vi "Remove_Current_Active_Hall_Call.vi"(8 "error in (no error)":errorcluster, 9 "Hall Calls Up/Down in":T1, 10 "Elevator in":T3, 11 "Elevator Fleet in":T10) -> (0 "error out":errorcluster, 1 "Hall Calls Up/Down out":T1, 2 "Elevator out":T3, 3 "Elevator Fleet out":T10)   [LabVIEW 2026]
uses:
  Controls/Elevator_Status.ctl
  Controls/Door_Status_Enum.ctl
  Controls/Occupy_Status.ctl
  Controls/Floor_Status.ctl
  Controls/Motion_Status_Enum.ctl
  Controls/Car_Calls_Status.ctl
  Controls/Hall_Calls_Status.ctl
  Controls/Elevator_Fleet.ctl
  Controls/Hall_Calls.ctl
  Controls/Hall_Floor.ctl
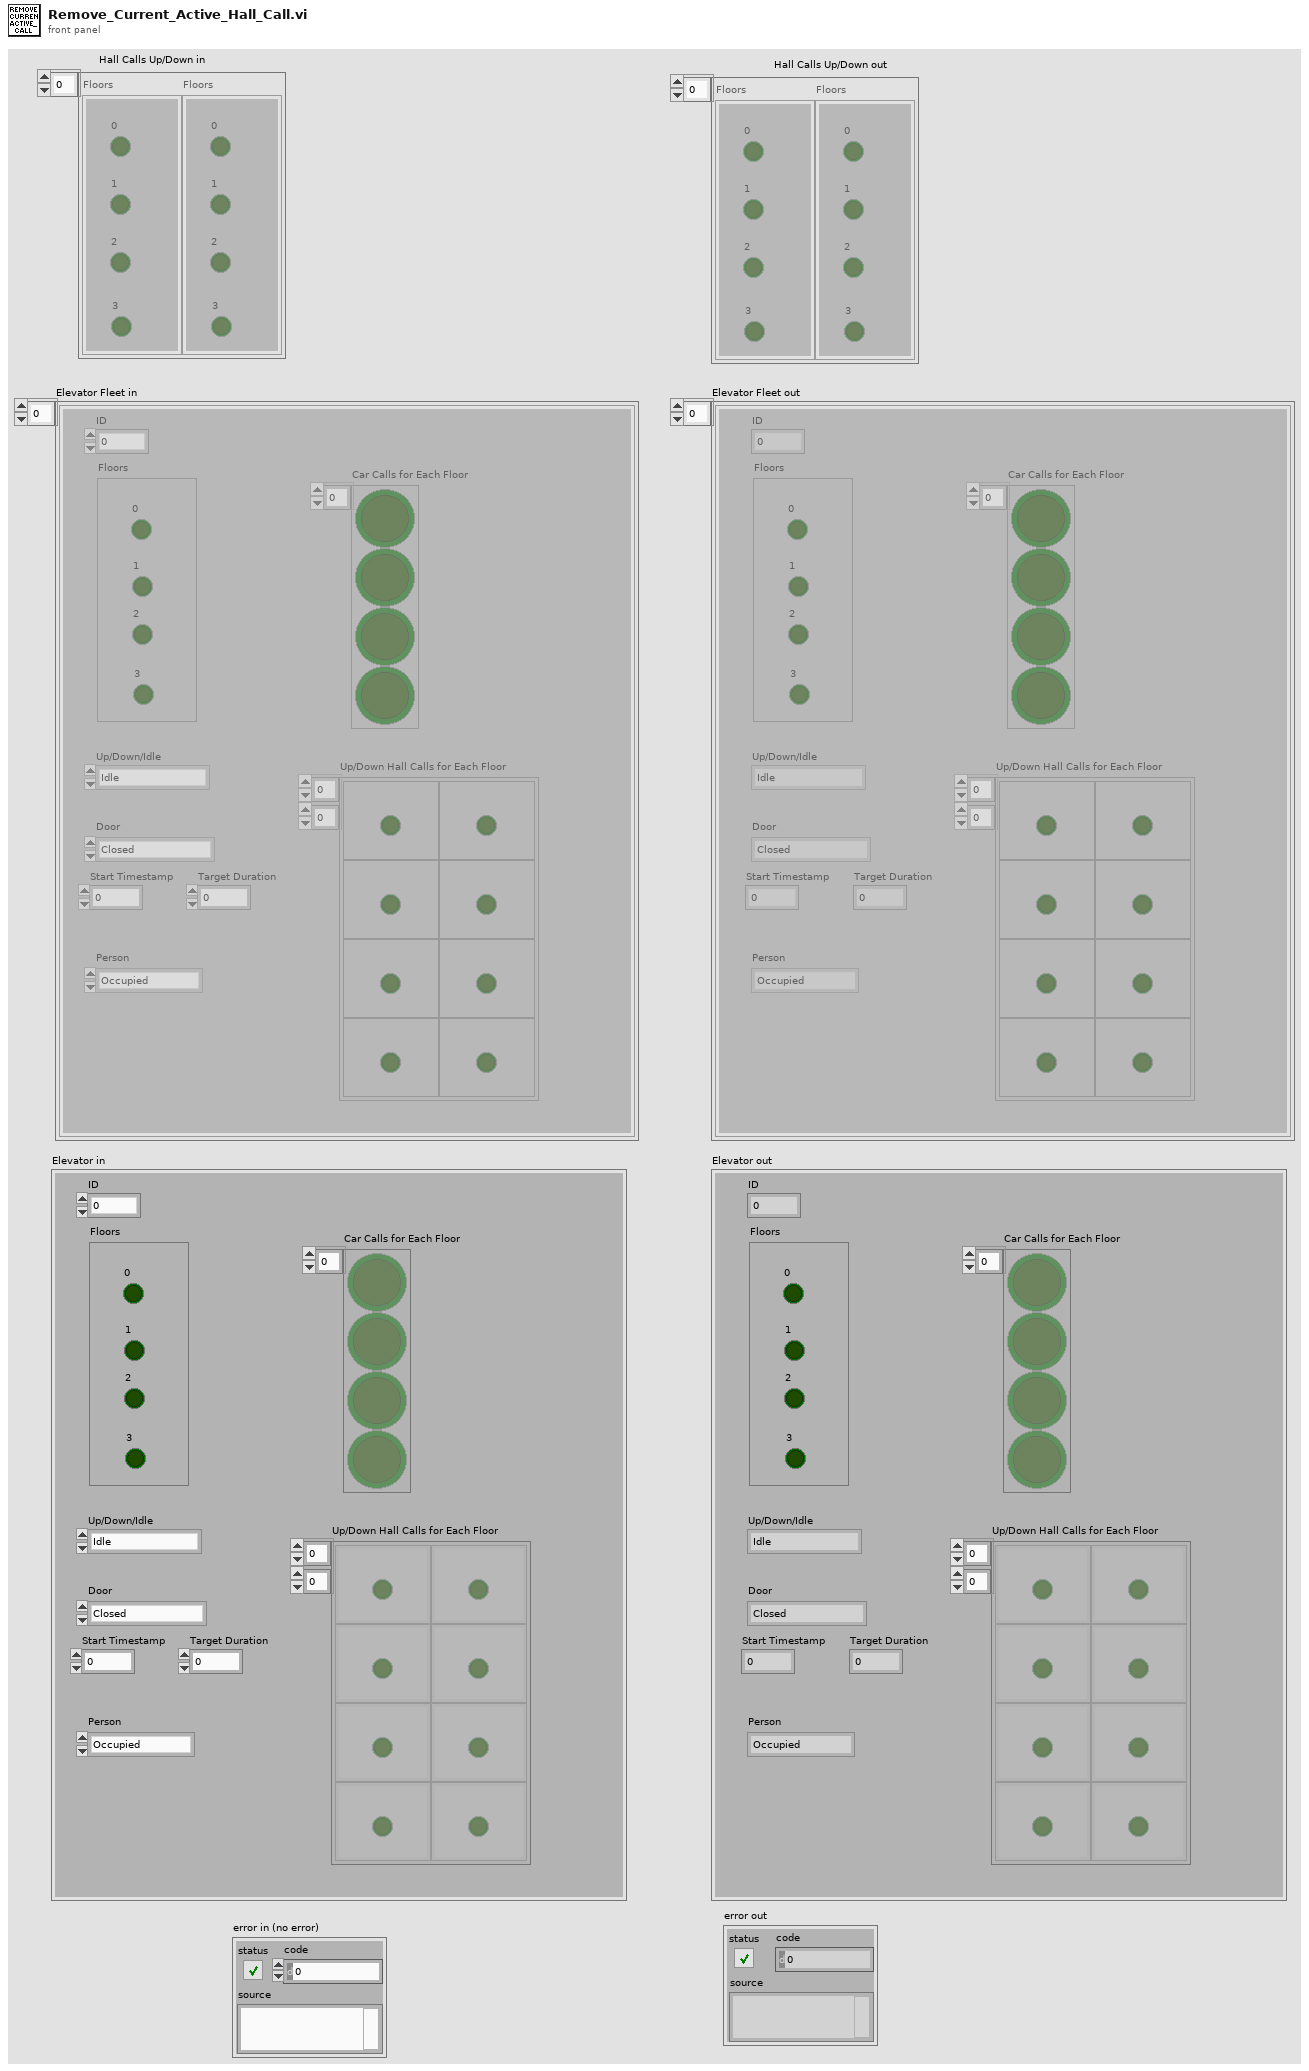
[diagram p1: front panel]
types:
  T1 = typedef "Hall_Calls.ctl" = T2[]
  T2 = typedef "Hall_Floor.ctl" = cluster{"0":bool, "1":bool, "2":bool, "3":bool}
  T3 = typedef "Elevator_Status.ctl" = cluster{"Door":T4, "Person":T5, "Floors":T6, "Up/Down/Idle":T7, "Car Calls for Each Floor":T8, "Up/Down Hall Calls for Each Floor":T9, "ID":i32, "Start Timestamp":u32, "Target Duration":dbl}
  T4 = typedef "Door_Status_Enum.ctl" = enum16{"Closed", "Open", "Opening", "Closing"}
  T5 = typedef "Occupy_Status.ctl" = enum16{"Occupied", "Empty"}
  T6 = typedef "Floor_Status.ctl" = cluster{"0":bool, "1":bool, "2":bool, "3":bool}
  T7 = typedef "Motion_Status_Enum.ctl" = enum16{"Idle", "Up", "Down"}
  T8 = typedef "Car_Calls_Status.ctl" = bool[]
  T9 = typedef "Hall_Calls_Status.ctl" = cluster{bool}[][]
  T10 = typedef "Elevator_Fleet.ctl" = T3[]
  T11 = enum16{"Check for Any Floor - Car Call", "Check for Specific Floor - Car Call", "Check for Any Floor - Hall Call", "Check for Specific Floor - Hall Call"}
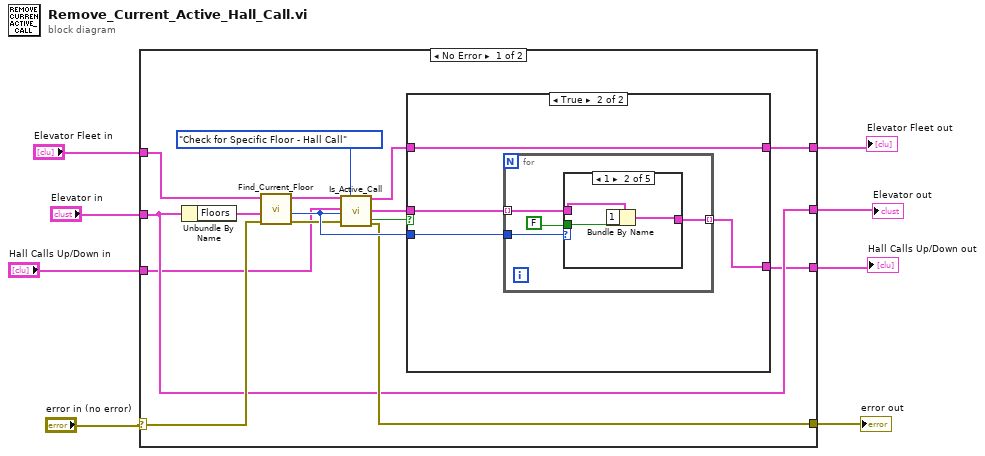
[diagram p0: block diagram]
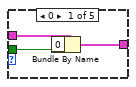
[diagram p3: hidden frame]
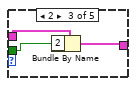
[diagram p4: hidden frame]
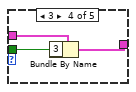
[diagram p5: hidden frame]
diagram:
  n1 = case shown="No Error" "error in (no error)" {
    selector: "error in (no error)" -> [w18 w50]
    tunnel: "Elevator in" -> [w12 w49]
    tunnel: "Elevator Fleet in" -> [w21 w48]
    tunnel: [w12 w49] -> w6
    tunnel: [w16 w50] -> w5
    tunnel: [w14 w48] -> w4
    tunnel: "Hall Calls Up/Down in" -> [w10 w47]
    tunnel: [w9 w47] -> w1
    frame No Error {
      n2 = Unbundle By Name(w12) -> ("Floors"=w19:T6)
      n3 = call "Find_Current_Floor.vi"("error in (no error)"=w18, "Floors"=w19, "Elevator Fleet in"=w21) -> ("error out"=w17:errorcluster, "Current Floor"=w22:i32, "Elevator Fleet out"=w20:T10)  [unwired: 5 in, 1 out]
      n4 = call "Is_Active_Call.vi"("Elevator Fleet in"=w20, "Enum"=T11."Check for Specific Floor - Hall Call", "Hall Calls Up/Down in"=w10, "Floor"=w22, "error in (no error)"=w17) -> ("Elevator Fleet out"=w15:T10, "Hall Calls Up/Down out"=w11:T1, "Active Call?"=w23:bool, "error out"=w16:errorcluster)  [unwired: 6 in, 1 out]
      n5 = case shown="True" w23 {
        tunnel: w22 -> [_ w27]
        tunnel: [w25 w29] -> w14
        tunnel: w15 -> [w25 w29]
        tunnel: w11 -> [w24 w28]
        tunnel: [w24 w26] -> w9
        frame False {
        }
        frame True {
          n6 = for {
            tunnel: w28 -> [w33] mode=indexing
            tunnel: w27 -> [w32]
            tunnel: [w30] -> w26 mode=indexing
            n7 = case shown="1" w32 {
              tunnel: w33 -> [w36 w39 w42 w45 w46]
              tunnel: FALSE -> [w35 w38 w41 w44 _]
              tunnel: [w34 w37 w40 w43 w46] -> w30
              frame 0 {
                n8 = Bundle By Name(cluster=w36, "0"=w35) -> (w34:T2)
              }
              frame 1 {
                n9 = Bundle By Name(cluster=w39, "1"=w38) -> (w37:T2)
              }
              frame 2 {
                n10 = Bundle By Name(cluster=w42, "2"=w41) -> (w40:T2)
              }
              frame 3 {
                n11 = Bundle By Name(cluster=w45, "3"=w44) -> (w43:T2)
              }
              frame Default {
              }
            }
          }
        }
      }
    }
    frame Error {
    }
  }
  "Elevator Fleet out" <- w4
  "Elevator out" <- w6
  "error out" <- w5
  "Hall Calls Up/Down out" <- w1
